vi "Set TMOD to Auto.vi"(8 "error in":errorcluster, 11 "SR PS3XX in":refnum<class "SR 3XX HVPS.lvclass">) -> (0 "error out":errorcluster, 3 "SR PS3XX out":refnum<class "SR 3XX HVPS.lvclass">)   [LabVIEW 2014, in "SR 3XX HVPS.lvclass"]
doc: "Set the trip mode to auto -the unit waits until the output voltage has fallen to 1/50 of its full scale value and then turns the high voltage back on. This is useful when dealing with loads that occasionally short circuit but recover after removing the high voltage."
uses:
  SR 3XX HVPS.lvclass
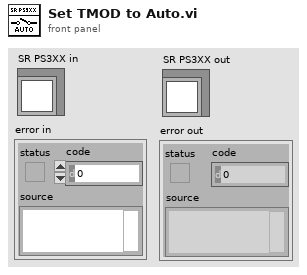
[diagram p1: front panel]
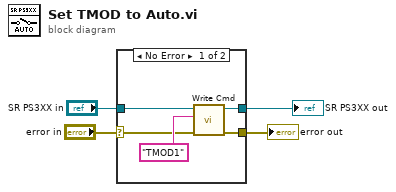
[diagram p0: block diagram]
diagram:
  n1 = case shown="No Error" "error in" {
    selector: "error in" -> [w7 w11]
    tunnel: [w5 w11] -> w3
    tunnel: [w6 w10] -> w1
    tunnel: "SR PS3XX in" -> [w8 w10]
    frame No Error {
      n2 = call "Write Cmd.vi"("error in"=w7, "Cmd"="TMOD1", "SR 3XX HVPS in"=w8) -> ("error out"=w5:errorcluster, "SR 3XX HVPS out"=w6:refnum<class "SR 3XX HVPS.lvclass">)  [unwired: 7 in]
    }
    frame Error {
    }
  }
  "error out" <- w3
  "SR PS3XX out" <- w1
